vi "entryDFSM_Configure.vi"(0 "NInstrSim":refnum<class "NInstrSim.lvclass">, 3 "DFSM_Internals in":T1, 5 "error in (no error)":errorcluster) -> (14 "dup NInstrSim":refnum<class "NInstrSim.lvclass">, 17 "DFSM_Internals out":T1, 19 "error out":errorcluster)   [LabVIEW 2009, in "HB_Device_Examples.lvlib" / "NInstrSim.lvclass"]
doc: "This VI performs <B>entry</B> action of DeviceFSM.Configure.\n\n<b>Hint:</b> This is a dynamic dispatch VI to be implemented by child classes."
uses:
  NInstrSim.lvclass
  lib.lib/HGF_LVC/HGF_StateCharts/HGF_DeviceFSM/HGF_DeviceFSM_Internals.ctl
  lib.lib/HGF_LVC/HGF_DeviceBaseClasses/HGF_VISADevice/HGF_VISADevice.lvclass
  lib.lib/HGF_LVC/HGF_DeviceBaseClasses/HGF_DeviceBaseClasses.lvlib
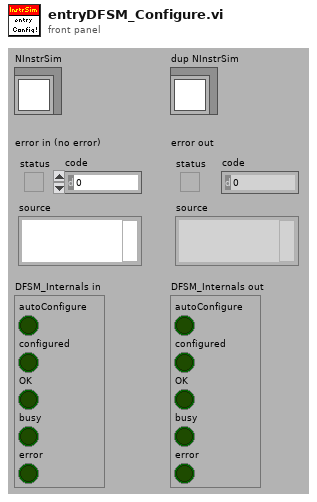
[diagram p1: front panel]
types:
  T1 = typedef "HGF_DeviceBaseClasses.lvlib/HGF_DeviceFSM_Internals.ctl" = cluster{"autoConfigure":bool, "configured":bool, "OK":bool, "busy":bool, "error":bool}
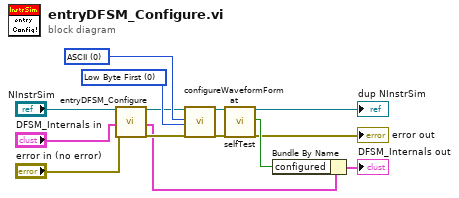
[diagram p0: block diagram]
diagram:
  w9 = u16 0 items=["Low Byte First", "High Byte First"] ("Byte Order (0:Low Byte First)")
  w10 = u16 0 items=["ASCII", "8-bit Unsigned Binary", "16-bit Signed Binary"] ("Waveform Format (0:ASCII)")
  n1 = call-parent "entryDFSM_Configure.vi"("HGF_DeviceBase"="NInstrSim", "DFSM_Internals in"="DFSM_Internals in", "error in (no error)"="error in (no error)") -> ("dup HGF_DeviceBase"=w6:refnum<class "NInstrSim.lvclass">, "DFSM_Internals out"=w4:T1, "error out"=w5:errorcluster)  [unwired: 14 out]
  n2 = call "configureWaveformFormat.vi"("NInstrSim"=w6, "Waveform Format (0:ASCII)"=w10, "Byte Order (0:Low Byte First)"=w9, "error in (no error)"=w5) -> ("dup NInstrSim"=w8:refnum<class "NInstrSim.lvclass">, "error out"=w7:errorcluster)  [unwired: 14 out]
  n3 = call-dynamic "selfTest.vi"("NInstrSim"=w8, "error in (no error)"=w7) -> ("dup NInstrSim"=→"dup NInstrSim":refnum<class "NInstrSim.lvclass">, "passed?"=w11:bool, "error out"=→"error out":errorcluster)  [unwired: 15 out]
  n4 = Bundle By Name(cluster=w4, "configured"=w11) -> (→"DFSM_Internals out":T1)
